vi "Configure Programmer.vi"(10 "Position":u32, 11 "Program RF MTS in":refnum<class "Program RF APP.lvclass">) -> (0 "Error out":errorcluster, 2 "Programmer out":refnum<class "Segger Flasher ARM.lvclass">)   [LabVIEW 2015, in "Program RF APP.lvclass"]
uses:
  Program RF APP.lvclass
  Classes/Programmer/Segger Flasher ARM/Class/Segger Flasher ARM.lvclass
  Classes/Application/Class/Application.lvclass
  Test Class/Test Class.lvclass
  <vilib>/Cree, Inc/Cree Test Framework/Classes/Base Objects/Base Class/Base Class/Base Class.lvclass
  Classes/Programmer/Programmer/Class/Programmer.lvclass
  Classes/Test Recipe/Class/Test Recipe.lvclass
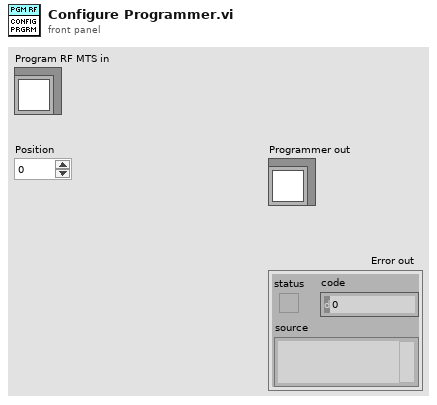
[diagram p1: front panel]
types:
  T1 = typedef "Application.lvlib/App Properties.lvclass/Class Properties -- Cluster.ctl" = cluster{"UUT Info":T2[], "Test Information":refnum<vi>, "Test Complete Event":refnum<user-event>, "Shop Floor System":refnum<class "Shop Floor System.lvclass">, "Gold Board":refnum<class "Golden Board.lvclass">, "Test Recipe":refnum<class "Test Recipe.lvclass">, "Instruments":refnum<class "Instrument.lvclass">[], "Mode":T3, "Test Results":cluster{"Pass":bool[], "Fail Codes":string[]}, "Station Config":refnum<class "Station Config.lvclass">}
  T2 = typedef "Application.lvlib/App Properties.lvclass/UUT Reference -- Cluster.ctl" = cluster{"Serial Number Reference":refnum<vi>, "Status Message Reference":refnum<vi>}
  T3 = typedef "Application.lvlib/Application.lvclass/Op Mode -- Enum.ctl" = u16
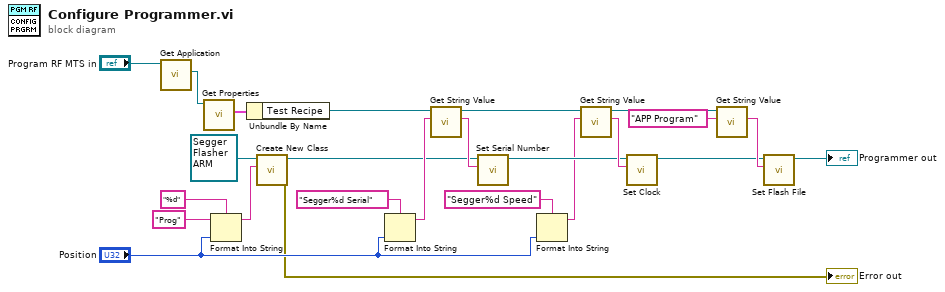
[diagram p0: block diagram]
diagram:
  n1 = call "Get Application.vi"("Test Class in"="Program RF MTS in") -> ("Application.lvlib:Application.lvclass"=w2:refnum<class "Application.lvclass">)  [unwired: 9 in, 1 out]
  n2 = call "Get Properties.vi"("Acrobat Template in"=w2) -> ("Class Properties"=w7:T1)  [unwired: 8 in, 2 out]
  n3 = Format Into String(format string="%d", initial string="Prog" ("Name"), "Position") -> (resulting string=w6:string)  [unwired: 1 in, 1 out]
  n4 = Unbundle By Name(w7) -> ("Test Recipe"=w10:refnum<class "Test Recipe.lvclass">)
  n5 = call <vilib>:"Create New Class.vi"("Name"=w6, "Base Class in"=refnum<class "Segger Flasher ARM.lvclass"> refnum ("Segger Flasher ARM.lvlib:Segger Flasher ARM.lvclass")) -> ("error out"=→"Error out":errorcluster, "Base Class out"=w8:refnum<class "Segger Flasher ARM.lvclass">)  [unwired: 8 in]
  n6 = Format Into String(format string="Segger%d Serial", "Position") -> (resulting string=w11:string)  [unwired: 2 in, 1 out]
  n7 = call "Get String Value.vi"("Name"=w11, "Test Recipe in"=w10) -> ("Value"=w12:string, "Test Recipe out"=w13:refnum<class "Test Recipe.lvclass">)  [unwired: 7 in, 1 out]
  n8 = call "Set Serial Number.vi"("Serial Number"=w12, "Programmer in"=w8) -> ("Programmer out"=w18:refnum<class "Segger Flasher ARM.lvclass">)  [unwired: 8 in, 1 out]
  n9 = Format Into String(format string="Segger%d Speed", "Position") -> (resulting string=w15:string)  [unwired: 2 in, 1 out]
  n10 = call "Get String Value.vi"("Name"=w15, "Test Recipe in"=w13) -> ("Value"=w19:string, "Test Recipe out"=w16:refnum<class "Test Recipe.lvclass">)  [unwired: 7 in, 1 out]
  n11 = call "Set Clock.vi"("Clock Speed"=w19, "Programmer in"=w18) -> ("Programmer out"=w20:refnum<class "Segger Flasher ARM.lvclass">)  [unwired: 8 in, 1 out]
  n12 = call "Get String Value.vi"("Name"="APP Program", "Test Recipe in"=w16) -> ("Value"=w21:string)  [unwired: 7 in, 2 out]
  n13 = call "Set Flash File.vi"("Flash File"=w21, "Programmer in"=w20) -> ("Programmer out"=→"Programmer out":refnum<class "Segger Flasher ARM.lvclass">)  [unwired: 8 in, 1 out]
